vi "数据库查询.vi"() -> ()   [LabVIEW 2018]
uses:
  <vilib>/addons/_office/_exclsub.llb/font.ctl
  <vilib>/Utility/NIReport.llb/Report Type.ctl
  <vilib>/addons/database/Connection.llb/DB Tools Open Connec (String).vi
  <vilib>/addons/_office/excel.llb/Excel Easy Table (str).vi
  <vilib>/Utility/NIReport.llb/NI_report.lvclass
  <vilib>/addons/database/NI_Database_API.lvlib
  <vilib>/addons/_office/NI_ReportGenerationToolkit.lvlib
  <vilib>/Utility/NIReport.llb/Excel/NI_Excel.lvclass
  <vilib>/ptbypt/NI_PtbyPt.lvlib
  FreeMem.dll
  <vilib>/Utility/NIReport.llb/NI_ReportGenerationCore.lvlib
panel:
  out "错误输出":errorcluster
  out "数字(0-1)":dbl
  out "Elapsed Time (s)":dbl caption="已用时间(s)"
  out "2天时间到释放资源":bool caption="结束"
  in  "Main Tab":enum32{""}(tab)
  in  "时间范围OFF":bool
  in  "结束日期":timestamp
  in  "起始日期":timestamp
  out "查询状态":string
  in  "总成码OFF":bool
  in  "总成码":string
  in  "二维码OFF":bool
  in  "二维码":string
  in  "数据类型":u16(ring) items=["ALL", "Online", "Offline", "Rework"]
  in  "产品状态":u16(ring) items=["ALL", "OK", "NG"]
  in  "导出":bool
  in  "退出":bool
  in  "查询":bool
  in  "另存为":bool
  out "查询结果":i32(listbox)
  # "2020-04-14_17:08"
  # "历史数据查询"
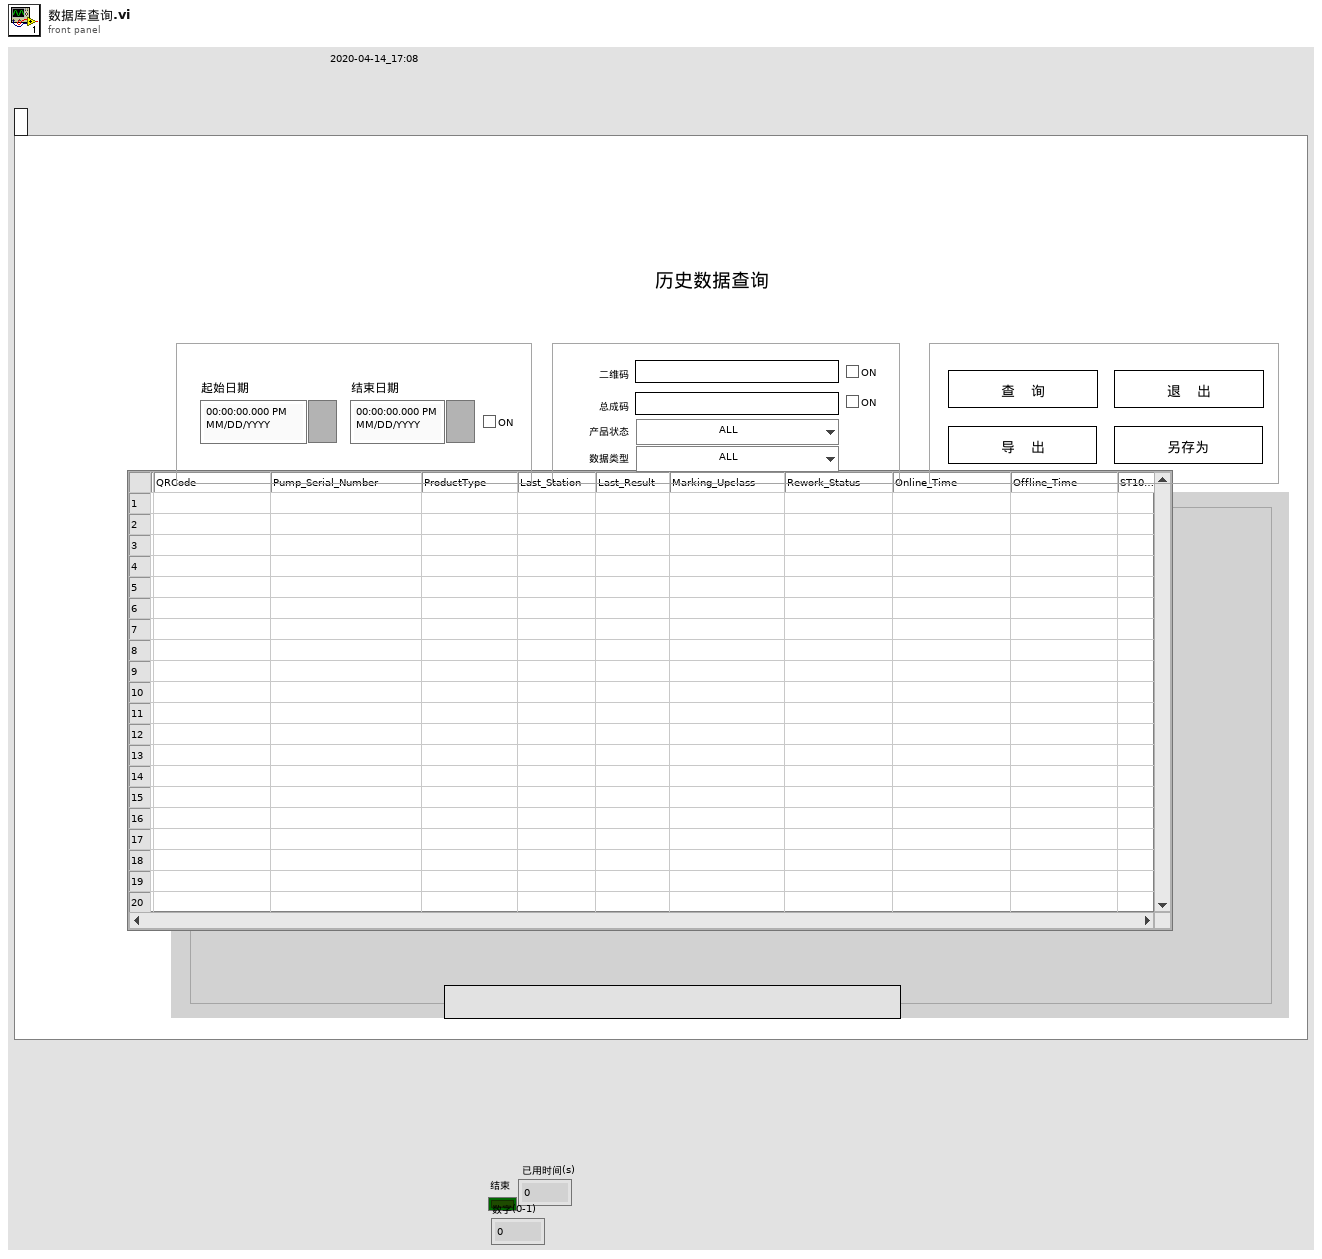
[diagram p1: front panel]
types:
  T1 = typedef "NI_ReportGenerationCore.lvlib/Report Type.ctl" = enum16{"HTML", "Word", "Excel"}
  T2 = typedef "NI_ReportGenerationToolkit.lvlib/font.ctl" = cluster{"font name":string, "font size":dbl, "bold":u16, "italic":u16, "underline":u16, "strike through":u16, "font color":u32}
  T3 = enum16{"maximized", "minimized", "normal", "no change"}
  T4 = enum32{"Invalid", "Standard", "Closed", "Hidden", "Minimized", "Maximized"}
  T5 = typedef "NI_Database_API.lvlib/Conn ObjectReference.ctl" = refnum<k1>
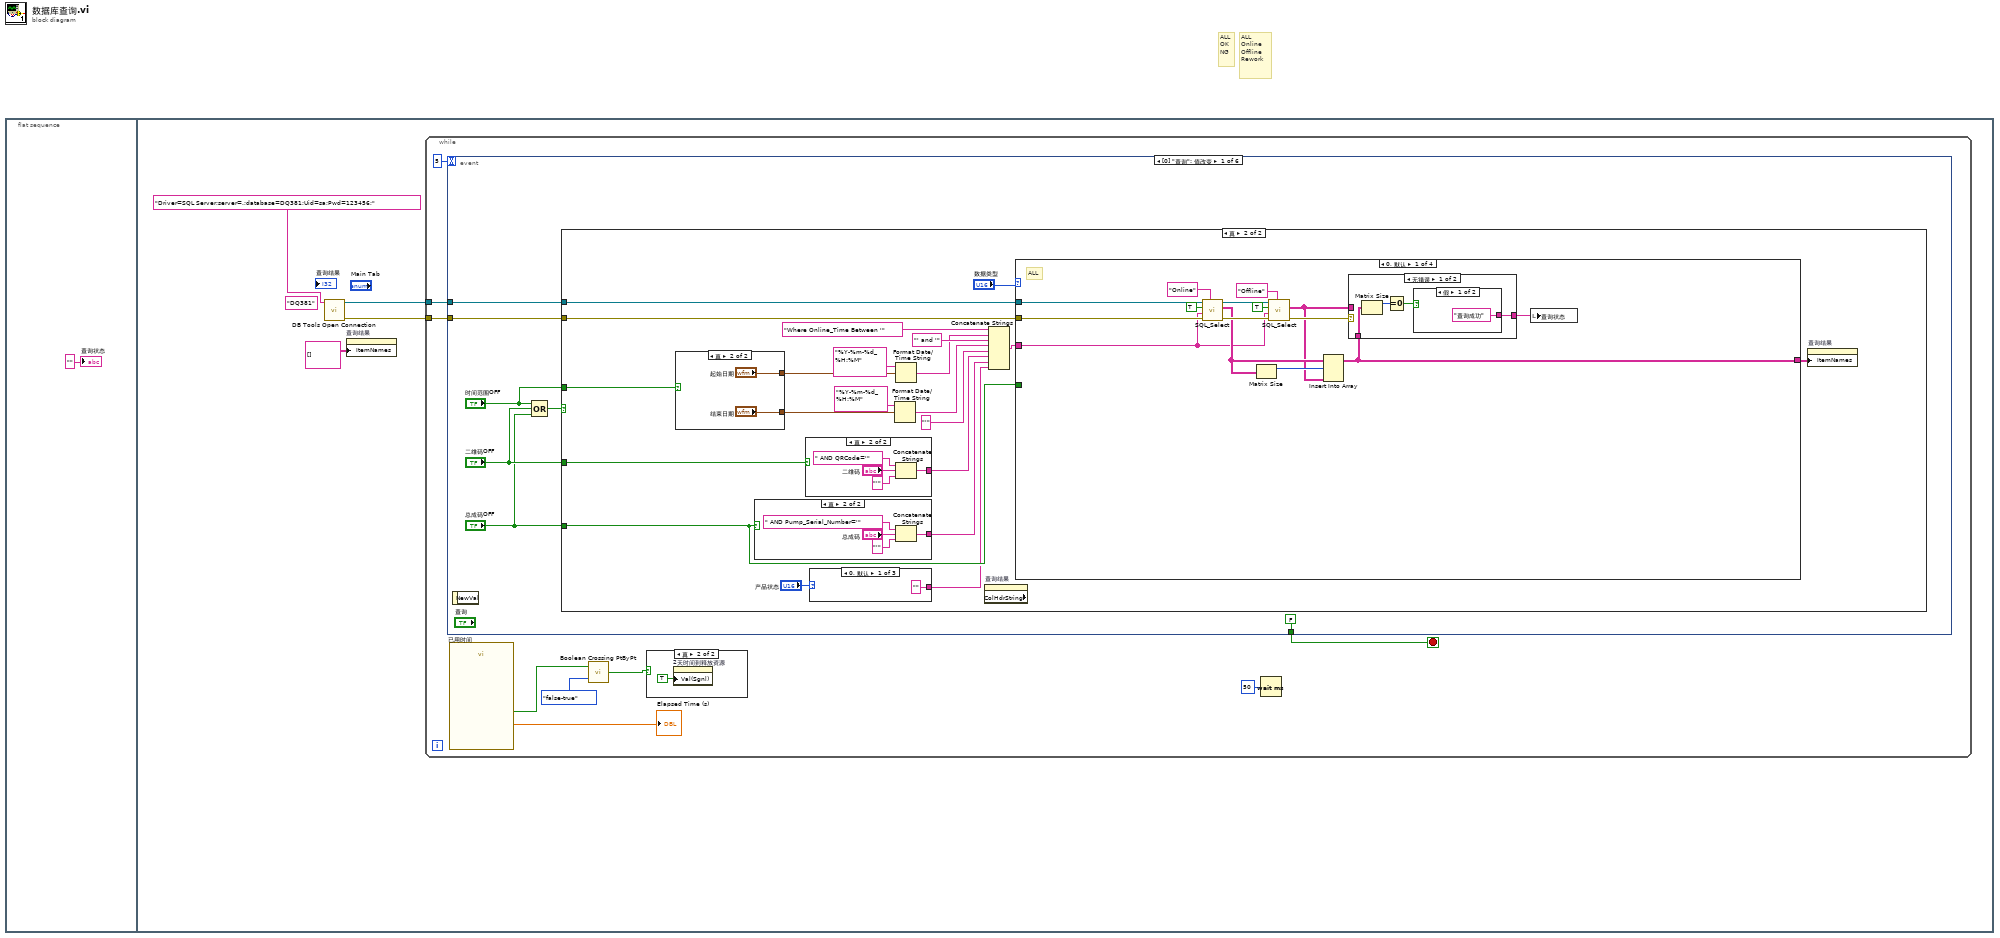
[diagram p0: block diagram]
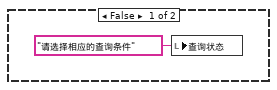
[diagram p3: hidden frame]
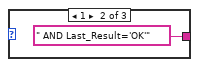
[diagram p4: hidden frame]
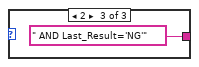
[diagram p5: hidden frame]
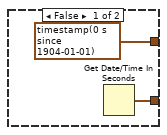
[diagram p6: hidden frame]
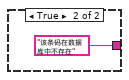
[diagram p7: hidden frame]
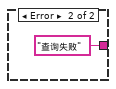
[diagram p8: hidden frame]
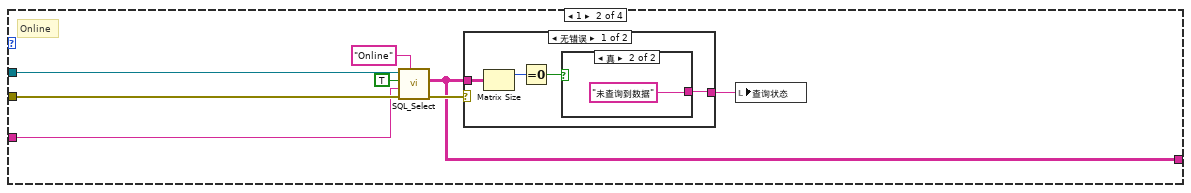
[diagram p9: hidden frame]
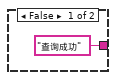
[diagram p10: hidden frame]
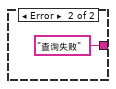
[diagram p11: hidden frame]
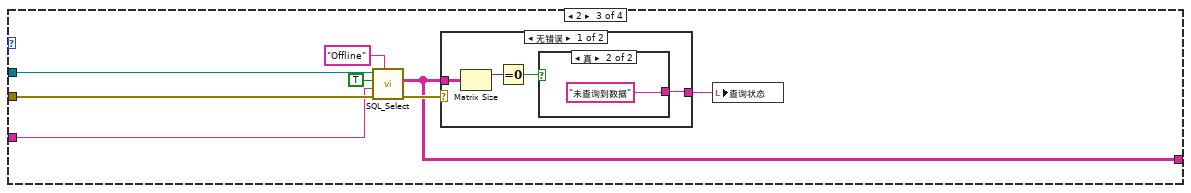
[diagram p12: hidden frame]
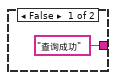
[diagram p13: hidden frame]
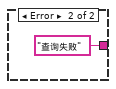
[diagram p14: hidden frame]
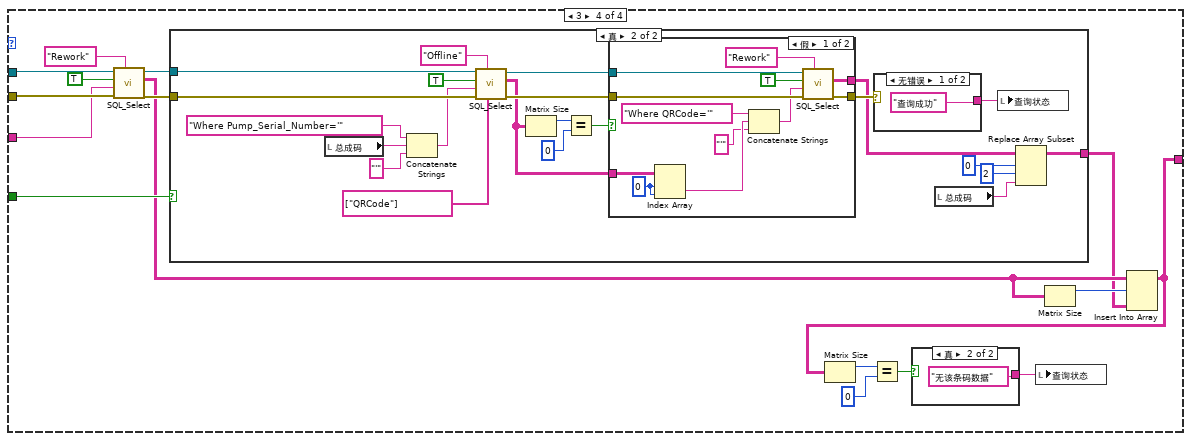
[diagram p15: hidden frame]
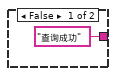
[diagram p16: hidden frame]
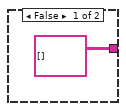
[diagram p17: hidden frame]
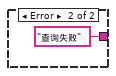
[diagram p18: hidden frame]
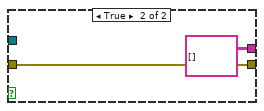
[diagram p19: hidden frame]
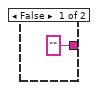
[diagram p20: hidden frame]
diagram:
  # "ALL\nOK\nNG"
  # "ALL\nOnline\nOffline\nRework"
  n1 = flat-sequence {
    frame #0 {
      "查询状态" <- "" ("查询状态")
    }
    frame #1 {
      (unwired) "DQ381"
      n2 = call-poly <vilib>:"DB Tools Open Connection.vi"("connection information"="Driver=SQL Server;server=.;database=DQ381;Uid=sa;Pwd=123456;") -> ("error out"=w4:errorcluster, "connection reference"=w5:T5)  [unwired: 7 in]
      n3 = property on="查询结果" class="MCListbox (严格)"("ItemNames"=string[][] [] ("项名")) -> ()  [unwired: 2 in, 2 out]
      n4 = while {
        tunnel: w5 -> [w14]
        tunnel: w4 -> [w13]
        stop <- w12 stop-if-true
        n5 = event shown="[0] \"查询\": 值改变" {
          selector: _ -> [_ _ _ _ _ _]
          dyn-events: _ -> [_ _ _ _ _ _]
          timeout: 5 -> [_ _ _ _ _ _]
          tunnel: w14 -> [w22 _ _ _ w233 _]
          tunnel: w13 -> [w21 _ _ _ w232 _]
          tunnel: [FALSE ("NewVal") _ FALSE ("NewVal") _ w234 _] -> w12
          event "查询": Value Change {
            n6 = event-data() -> ()  [unwired: 1 in, 1 out]
            n7 = Compound Arithmetic op=OR("时间范围OFF", "二维码OFF", "总成码OFF") -> (w17:bool)
            n8 = case shown="真" w17 {
              tunnel: w22 -> [_ w44]
              tunnel: w21 -> [_ w43]
              tunnel: "二维码OFF" -> [_ w28]
              tunnel: "总成码OFF" -> [_ w27]
              tunnel: "时间范围OFF" -> [_ w26]
              frame False {
                n9 = local write "查询状态"("请选择相应的查询条件" ("查询状态")) -> ()
              }
              frame True {
                n10 = case shown="真" w26 {
                  tunnel: [timestamp(0 s since 1904-01-01) ("起始日期") "起始日期"] -> w39
                  tunnel: [w48 "结束日期"] -> w36
                  frame False {
                    n11 = Get Date/Time In Seconds() -> (seconds since 1Jan1904=w48:timestamp)
                  }
                  frame True {
                  }
                }
                n12 = case shown="真" w27 {
                  tunnel: ["" w163] -> w30
                  frame False {
                  }
                  frame True {
                    n13 = Concatenate Strings(" AND Pump_Serial_Number='" ("字符串"), "总成码", "'" ("字符串")) -> (w163:string)
                  }
                }
                n14 = case shown="真" w28 {
                  tunnel: ["" w167] -> w34
                  frame False {
                  }
                  frame True {
                    n15 = Concatenate Strings(" AND QRCode='" ("字符串"), "二维码", "'" ("字符串")) -> (w167:string)
                  }
                }
                n16 = case shown="0, 默认" "产品状态" {
                  tunnel: ["" " AND Last_Result='OK'" ("字符串") " AND Last_Result='NG'" ("字符串")] -> w24
                  frame 0, Default {
                  }
                  frame 1 {
                  }
                  frame 2 {
                  }
                }
                n17 = Format Date/Time String(time format string (%c)="%Y-%m-%d_%H:%M" ("时间格式字符串(%c)"), seconds (now)=w36) -> (date/time string=w35:string)  [unwired: 1 in]
                n18 = Format Date/Time String(time format string (%c)="%Y-%m-%d_%H:%M" ("时间格式字符串(%c)"), seconds (now)=w39) -> (date/time string=w38:string)  [unwired: 1 in]
                n19 = property on="查询结果" class="MCListbox (严格)" props=["ColHdrString"]() -> ()  [unwired: 2 in, 3 out]
                n20 = Concatenate Strings("Where Online_Time Between '" ("查询语句"), w38, "' and '" ("字符串"), w35, "'" ("字符串"), w34, w30, w24) -> (w33:string)
                n21 = case shown="0, 默认" "数据类型" {
                  tunnel: w44 -> [w66 w77 w92 w117]
                  tunnel: w43 -> [w65 w76 w91 w116]
                  tunnel: w33 -> [w56 w75 w90 w115]
                  tunnel: [w52 w74 w89 w108] -> w32
                  tunnel: w27 -> [_ _ _ w114]
                  frame 0, Default {
                    # "ALL"
                    n22 = call "SQL_Select.vi"("表名"="Online", "error in (no error)"=w65, "查询语句"=w56, "查询条件"=TRUE, "connection reference"=w66) -> ("error out"=w61:errorcluster, "数据"=w58:string[][], "connection reference out"=w60:T5)  [unwired: 4 in]
                    n23 = Matrix Size(0:w58) -> (1:w57:i32)  [unwired: 1 out]
                    n24 = call "SQL_Select.vi"("表名"="Offline", "error in (no error)"=w61, "查询语句"=w56, "查询条件"=TRUE, "connection reference"=w60) -> ("error out"=w55:errorcluster, "数据"=w53:string[][])  [unwired: 4 in, 1 out]
                    n25 = Insert Into Array(array=w58, index (row)=w57, new element=w53) -> (w52:string[][])  [unwired: 1 in]
                    n26 = case shown="无错误" w55 {
                      tunnel: [w68 "查询失败"] -> w54
                      tunnel: w53 -> [_ _]
                      tunnel: w52 -> [w67 _]
                      frame No Error {
                        n27 = Matrix Size(0:w67) -> (1:w70:i32)  [unwired: 1 out]
                        n28 = Equal To 0?(x=w70) -> (x = 0?=w69:bool)
                        n29 = case shown="假" w69 {
                          tunnel: ["查询成功" "该条码在数据库中不存在"] -> w68
                          frame False {
                          }
                          frame True {
                          }
                        }
                      }
                      frame Error {
                      }
                    }
                    n30 = local write "查询状态"(w54) -> ()
                  }
                  frame 1 {
                    # "Online"
                    n31 = call "SQL_Select.vi"("表名"="Online", "error in (no error)"=w76, "查询语句"=w75, "查询条件"=TRUE, "connection reference"=w77) -> ("error out"=w79:errorcluster, "数据"=w74:string[][])  [unwired: 4 in, 1 out]
                    n32 = case shown="无错误" w79 {
                      tunnel: [w83 "查询失败"] -> w78
                      tunnel: w74 -> [w82 _]
                      frame No Error {
                        n33 = Matrix Size(0:w82) -> (1:w85:i32)  [unwired: 1 out]
                        n34 = Equal To 0?(x=w85) -> (x = 0?=w84:bool)
                        n35 = case shown="真" w84 {
                          tunnel: ["查询成功" "未查询到数据"] -> w83
                          frame False {
                          }
                          frame True {
                          }
                        }
                      }
                      frame Error {
                      }
                    }
                    n36 = local write "查询状态"(w78) -> ()
                  }
                  frame 2 {
                    n37 = call "SQL_Select.vi"("表名"="Offline", "error in (no error)"=w91, "查询语句"=w90, "查询条件"=TRUE, "connection reference"=w92) -> ("error out"=w94:errorcluster, "数据"=w89:string[][])  [unwired: 4 in, 1 out]
                    n38 = case shown="无错误" w94 {
                      tunnel: [w98 "查询失败"] -> w93
                      tunnel: w89 -> [w97 _]
                      frame No Error {
                        n39 = Matrix Size(0:w97) -> (1:w100:i32)  [unwired: 1 out]
                        n40 = Equal To 0?(x=w100) -> (x = 0?=w99:bool)
                        n41 = case shown="真" w99 {
                          tunnel: ["查询成功" "未查询到数据"] -> w98
                          frame False {
                          }
                          frame True {
                          }
                        }
                      }
                      frame Error {
                      }
                    }
                    n42 = local write "查询状态"(w93) -> ()
                  }
                  frame 3 {
                    n43 = call "SQL_Select.vi"("表名"="Rework", "error in (no error)"=w116, "查询语句"=w115, "查询条件"=TRUE, "connection reference"=w117) -> ("error out"=w113:errorcluster, "数据"=w110:string[][], "connection reference out"=w112:T5)  [unwired: 4 in]
                    n44 = case shown="真" w114 {
                      tunnel: w113 -> [_ w144]
                      tunnel: w112 -> [_ w143]
                      tunnel: [string[][] [] ("数据") w123] -> w109
                      frame False {
                      }
                      frame True {
                        n45 = local read "总成码"() -> (w138:string)
                        n46 = Concatenate Strings("Where Pump_Serial_Number='" ("查询语句"), w138, "'" ("字符串")) -> (w137:string)
                        n47 = call "SQL_Select.vi"("要读取的列名"=string[] ["QRCode"], "表名"="Offline", "error in (no error)"=w144, "查询语句"=w137, "查询条件"=TRUE, "connection reference"=w143) -> ("error out"=w131:errorcluster, "数据"=w130:string[][], "connection reference out"=w132:T5)  [unwired: 3 in]
                        n48 = Matrix Size(0:w130) -> (1:w135:i32)  [unwired: 1 out]
                        n49 = Equal?(x=w135, y=0) -> (x = y?=w133:bool)
                        n50 = case shown="假" w133 {
                          tunnel: w132 -> [w158 _]
                          tunnel: w131 -> [w157 w160]
                          tunnel: [w154 string[][] [] ("数据")] -> w127
                          tunnel: [w153 w160] -> w128
                          tunnel: w130 -> [w150 _]
                          frame False {
                            w149 = 0 ("索引 (行)")
                            n51 = Index Array(array=w150, index (row)=w149, index (col)=w149) -> (element=w148:string)
                            n52 = Concatenate Strings("Where QRCode='" ("查询语句"), w148, "'" ("字符串")) -> (w152:string)
                            n53 = call "SQL_Select.vi"("表名"="Rework", "error in (no error)"=w157, "查询语句"=w152, "查询条件"=TRUE, "connection reference"=w158) -> ("error out"=w153:errorcluster, "数据"=w154:string[][])  [unwired: 4 in, 1 out]
                          }
                          frame True {
                          }
                        }
                        n54 = case shown="无错误" w128 {
                          tunnel: ["查询成功" "查询失败"] -> w129
                          frame No Error {
                          }
                          frame Error {
                          }
                        }
                        n55 = local read "总成码"() -> (w124:string)
                        n56 = local write "查询状态"(w129) -> ()
                        n57 = Replace Array Subset(array=w127, new element=w124, index (row)=0 ("索引 (行)"), index (col)=2 ("禁用的索引 (列)")) -> (w123:string[][])
                      }
                    }
                    n58 = Matrix Size(0:w110) -> (1:w111:i32)  [unwired: 1 out]
                    n59 = Insert Into Array(array=w110, index (row)=w111, new element=w109) -> (w108:string[][])  [unwired: 1 in]
                    n60 = Matrix Size(0:w108) -> (1:w107:i32)  [unwired: 1 out]
                    n61 = Equal?(x=w107, y=0) -> (x = y?=w104:bool)
                    n62 = case shown="真" w104 {
                      tunnel: ["查询成功" "无该条码数据"] -> w105
                      frame False {
                      }
                      frame True {
                      }
                    }
                    n63 = local write "查询状态"(w105) -> ()
                  }
                }
                n64 = property on="查询结果" class="MCListbox (严格)"("ItemNames"=w32) -> ()  [unwired: 2 in, 2 out]
              }
            }
          }
          event Timeout {
            n65 = event-data() -> ()  [unwired: 1 in, 3 out]
          }
          event "另存为": Value Change {
            n66 = event-data() -> ()  [unwired: 1 in, 1 out]
            n67 = property on="查询结果" class="MCListbox (严格)"() -> ("ItemNames"=w176:string[][])  [unwired: 2 in, 2 out]
            n68 = property on="查询结果" class="MCListbox (严格)"() -> ("ColHdrString"=w179:string[])  [unwired: 2 in, 2 out]
            n69 = for {
              tunnel: w176 -> [w184] mode=indexing
              tunnel: [w181] -> w174 mode=indexing
              n70 = Delete From Array(array=w184, length=1 ("长度"), index=0 ("索引")) -> (array with subset deleted=w181:string[])  [unwired: 1 out]
            }
            n71 = Delete From Array(array=w179, length=1 ("长度"), index=0 ("索引")) -> (array with subset deleted=w173:string[])  [unwired: 1 out]
            n72 = Insert Into Array(array=w174, index (row)=0 ("索引"), new element=w173) -> (w172:string[][])  [unwired: 1 in]
            n73 = call "Save to EXCEL.vi"("text data"=w172) -> ("error out"=w171:errorcluster)  [unwired: 10 in]
            n74 = call <vilib>:"Clear Errors.vi"("error in (no error)"=w171) -> ()  [unwired: 5 in, 2 out]
          }
          event "导出": Value Change {
            (unwired) path "D:/Model/EXCEL.xlsx" ("template (empty)")
            w209 = 1 items=["left", "center", "right"] ("horizontal alignment (left)")
            n75 = event-data() -> ()  [unwired: 1 in, 3 out]
            n76 = property on="查询结果" class="MCListbox (严格)"() -> ("ItemNames"=w214:string[][])  [unwired: 2 in, 2 out]
            n77 = call <vilib>:"Check if File or Folder Exists.vi"("path"=path "D:/Data_Storage/Data" ("文件路径（使用对话框）")) -> ("error out"=w197:errorcluster, "file or folder exists?"=w199:bool, "dup path"=w198:path)  [unwired: 8 in]
            n78 = property on="查询结果" class="MCListbox (严格)"() -> ("ColHdrString"=w217:string[])  [unwired: 2 in, 2 out]
            n79 = for {
              tunnel: w214 -> [w229] mode=indexing
              tunnel: [w226] -> w212 mode=indexing
              n80 = Delete From Array(array=w229, length=1 ("长度"), index=0 ("索引")) -> (array with subset deleted=w226:string[])  [unwired: 1 out]
            }
            n81 = Format Date/Time String(time format string (%c)="%Y%m%d%H%M%S" ("时间格式字符串(%c)")) -> (date/time string=w195:string)  [unwired: 2 in]
            n82 = case shown="假" w199 {
              tunnel: w198 -> [w223 w225]
              tunnel: [w222 w225] -> w193
              tunnel: w197 -> [w221 w224]
              tunnel: [w220 w224] -> _
              frame False {
                n83 = Create Folder(path (use dialog)=w223, error in=w221) -> (created path=w222:path, error out=w220:errorcluster)  [unwired: 1 in, 1 out]
              }
              frame True {
              }
            }
            n84 = Delete From Array(array=w217, length=1 ("长度"), index=0 ("索引")) -> (array with subset deleted=w211:string[])  [unwired: 1 out]
            n85 = Concatenate Strings(w195, ".xlsx" ("字符串")) -> (w192:string)
            n86 = Build Path(base path=w193, name or relative path=w192) -> (appended path=w191:path)
            n87 = Insert Into Array(array=w212, index (row)=0 ("索引"), new element=w211) -> (w201:string[][])  [unwired: 1 in]
            n88 = call <vilib>:"Create Report.vi"("window state (normal)"=T3."no change", "report type"=Report_Type."Excel") -> ("report out"=w186:refnum<class "NI_report.lvclass">, "error out"=w185:errorcluster)  [unwired: 12 in]
            n89 = call-poly <vilib>:"Excel Easy Table.vi"("report in"=w186, "font"=T2 {"font name"="", "font size"=12.0, "bold"=0, "italic"=0, "underline"=0, "strike through"=0, "font color"=16777216}, "start (0, 0)"=cluster{"row":i32, "column":i32} {"row"=0, "column"=0}, "text data"=w201, "error in (no error)"=w185) -> ("report out"=w207:refnum<class "NI_report.lvclass">, "error out"=w208:errorcluster)  [unwired: 6 in, 3 out]
            n90 = call <vilib>:"Excel Set Cell Alignment.vi"("report in"=w207, "horizontal alignment (left)"=w209, "error in (no error)"=w208) -> ("report out"=w202:refnum<class "NI_report.lvclass">, "error out"=w205:errorcluster)  [unwired: 11 in]
            n91 = call-dynamic "Save Report to File.vi"("report in"=w202, "report file path"=w191, "error in (no error)"=w205) -> ("report out"=w203:refnum<class "NI_report.lvclass">, "error out"=w204:errorcluster)  [unwired: 11 in]
            n92 = call-dynamic "Dispose Report.vi"("report in"=w203, "error in (no error)"=w204) -> ("error out"=w190:errorcluster)  [unwired: 13 in]
            n93 = case shown="错误" w190 {
              tunnel: ["导出成功" "导出失败"] -> w189
              frame No Error {
              }
              frame Error {
              }
            }
            n94 = call <vilib>:"Clear Errors.vi"("error in (no error)"=w190) -> ()  [unwired: 5 in, 2 out]
            n95 = local write "查询状态"(w189) -> ()
          }
          event "退出": Value Change {
            n96 = event-data() -> ("NewVal"=w234:bool)  [unwired: 1 in]
            n97 = call <vilib>:"DB Tools Close Connection.vi"("error in (no error)"=w232, "connection reference"=w233) -> ()  [unwired: 5 in, 1 out]
            n98 = control-ref of="本VI"() -> (w231:refnum<vi>)
            n99 = property class="VI"(reference=w231, "FP.State"=T4."Closed" ("前面板窗口:状态")) -> ()  [unwired: 1 in, 2 out]
          }
          event "2天时间到释放资源": Value Change {
            n100 = event-data() -> ()  [unwired: 1 in, 3 out]
            n101 = Random Number (0-1)() -> (number: 0 to 1=→"数字(0-1)":dbl)
            n102 = dll-call lib="PTH2abs E$èå·åæ³°ç§æè¡ä»½æéå¬å¸é¡¹ç®éº¦æ ¼çº³ç¨åºDQ381DQ501æ¹é -YT20-031381381-LV2018Project-20210928ProjectFreeMem.dll" fn="FreeMem"() -> (error out=→"错误输出":errorcluster)  [unwired: 4 in, 1 out]
          }
        }
        n103 = call "已用时间"() -> ("Elapsed Time (s)"=→"Elapsed Time (s)":dbl, "Time has Elapsed"=w8:bool)  [unwired: 12 in, 6 out]
        n104 = call <vilib>:"Boolean Crossing PtByPt.vi"("direction"=enum16{"either", "false-true", "true-false"}."false-true", "input"=w8) -> ("crossing"=w7:bool)  [unwired: 1 in]
        n105 = case shown="真" w7 {
          frame False {
          }
          frame True {
            n106 = property on="2天时间到释放资源" class="Bool (严格)"("Val(Sgnl)"=TRUE ("值(信号)")) -> ()  [unwired: 2 in, 2 out]
          }
        }
        n107 = Wait (ms)(milliseconds to wait=u32 50 ("等待时间（毫秒）")) -> ()  [unwired: 1 out]
      }
    }
  }
